vi "Collapse Tree.vi"(8 "error in":errorcluster, 11 "Report Viewer in":refnum<class "Report Viewer.lvclass">) -> (0 "error out":errorcluster, 3 "Report Viewer out":refnum<class "Report Viewer.lvclass">)   [LabVIEW 2019, in "Report Viewer.lvlib" / "Report Viewer.lvclass"]
uses:
  Library/Report Viewer.lvclass
  Library/Report Viewer.lvclass/Report Viewer.ctl
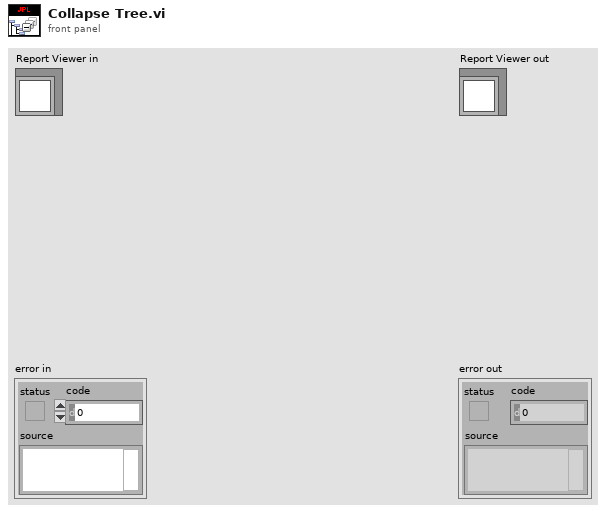
[diagram p1: front panel]
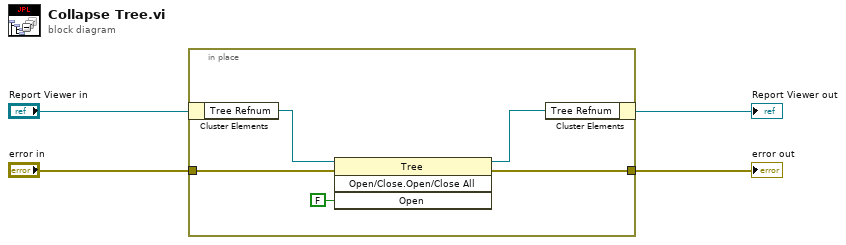
[diagram p0: block diagram]
diagram:
  n1 = in-place {
    in-place-border: [w6] -> w2
    in-place-border: "error in" -> [w5]
    n2 = in-place-cluster #1("Report Viewer in") -> ("Tree Refnum"=w8:refnum<vi>)
    n3 = invoke class="Tree" method="Open/Close.Open/Close All"(reference=w8, error in=w5, "Open"=FALSE ("Open?")) -> (reference out=w7:refnum<vi>, error out=w6:errorcluster)  [unwired: 1 in, 2 out]
    n4 = in-place-cluster #1("Tree Refnum"=w7) -> (→"Report Viewer out":refnum<class "Report Viewer.lvclass">)
  }
  "error out" <- w2
